vi "Auto Number Add.vi"(8 "error in (no error)":errorcluster, 10 "Auto Number Record":T1, 11 "Connection Refnum":T2) -> (0 "error out":errorcluster, 3 "Connection Refnum":T2)   [LabVIEW 2011]
uses:
  Summitek EXT/ODBC/SQL Controls/Connection Refnum.ctl
  Auto Number Record.ctl
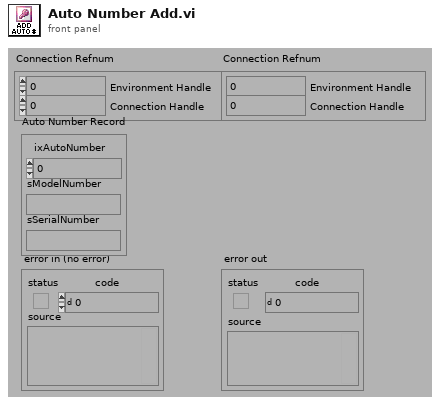
[diagram p1: front panel]
types:
  T1 = typedef "Auto Number Record.ctl" = cluster{"ixAutoNumber":i32, "sModelNumber":string, "sSerialNumber":string}
  T2 = typedef "Connection Refnum.ctl" = cluster{"Environment Handle":i32, "Connection Handle":i32}
  T3 = typedef "Statement Refnum.ctl" = cluster{"Statement Handle":i32, "Parameter Number":u16}
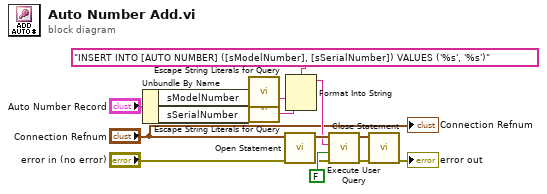
[diagram p0: block diagram]
diagram:
  n1 = Unbundle By Name("Auto Number Record") -> ("sModelNumber"=w6:string, "sSerialNumber"=w5:string)
  n2 = call "Escape String Literals for Query.vi"("String"=w6) -> ("escaped String"=w4:string)  [unwired: 1 in, 13 out]
  n3 = call "Escape String Literals for Query.vi"("String"=w5) -> ("escaped String"=w3:string)  [unwired: 1 in, 13 out]
  n4 = call "Open Statement.vi"("error in (no error)"="error in (no error)", "Connection Refnum"="Connection Refnum") -> ("error out"=w12:errorcluster, "Statement Refnum"=w11:T3)  [unwired: 4 out]
  n5 = Format Into String(format string="INSERT INTO [AUTO NUMBER] ([sModelNumber], [sSerialNumber]) VALUES ('%s', '%s')", w4, w3) -> (resulting string=w9:string)  [unwired: 2 in, 1 out]
  n6 = call "Execute User Query.vi"("error in (no error)"=w12, "Return Data? (f)"=FALSE, "User Query"=w9, "Statement Refnum"=w11) -> ("error out"=w13:errorcluster, "Statement Refnum"=w14:T3)  [unwired: 2 out]
  n7 = call "Close Statement.vi"("error in (no error)"=w13, "Statement Refnum"=w14) -> ("error out"=→"error out":errorcluster)  [unwired: 5 out]
  "Connection Refnum" <- "Connection Refnum"
